vi "SPC_get_eeprom_data.vi"(8 "Error In":errorcluster, 10 "Module No":i16 min=0 max=31 step=1, 11 "DLL Path":path) -> (0 "Error Out":errorcluster, 2 "Module No":i16 min=0 max=7 step=1, 3 "DLL Path":path, 4 "Revision [U8]":u8[](array[numeric]), 5 "SPC EEPROM Data":T1={"module_type[16]"="                ", "serial_no[16]"="                ", "date[16]"="                ", "SPC adjust parameters"={"vrt1"=64, "vrt2"=128, "vrt3"=192, "dith_g"=128, "gain_1"=1.0, "gain_2"=1.0, "gain_4"=1.0, "gain_8"=1.0, "tac_r0"=1.0, "tac_r1"=1.0, "tac_r2"=1.0, "tac_r4"=1.0, "tac_r8"=1.0, "sync_div"=0}} {"SPC adjust parameters"."sync_div" min=0 max=2; "SPC adjust parameters"."tac_r8" format="%.2f"; "SPC adjust parameters"."tac_r4" format="%.2f"; "SPC adjust parameters"."tac_r2" format="%.2f"; "SPC adjust parameters"."tac_r1" format="%.2f"; "SPC adjust parameters"."tac_r0" format="%.2f"; "SPC adjust parameters"."gain_8" format="%.2f"; "SPC adjust parameters"."gain_4" format="%.2f"; "SPC adjust parameters"."gain_2" format="%.2f"; "SPC adjust parameters"."gain_1" format="%.2f"}, 6 "Revision":i16)   [LabVIEW 2023]
doc: "The structure \"eep_data\" is filled with the contents of EEPROM of SPC module ‘mod_no’. \nThe EEPROM contains production data and adjust parameters of the module. The structure \"SPC_EEP_Data\" is defined in the file spcm_def.h.\nNormally, the EEPROM data need not be read explicitly because the EEPROM is read during SPC_init and the module type information and the adjust values are taken into account when the SPC module registers are loaded.\n\ninfo@becker-hickl.com"
uses:
  SPC_Controls/SPC_eep_data.ctl
  SPC_Controls/SPC_adjust_para.ctl
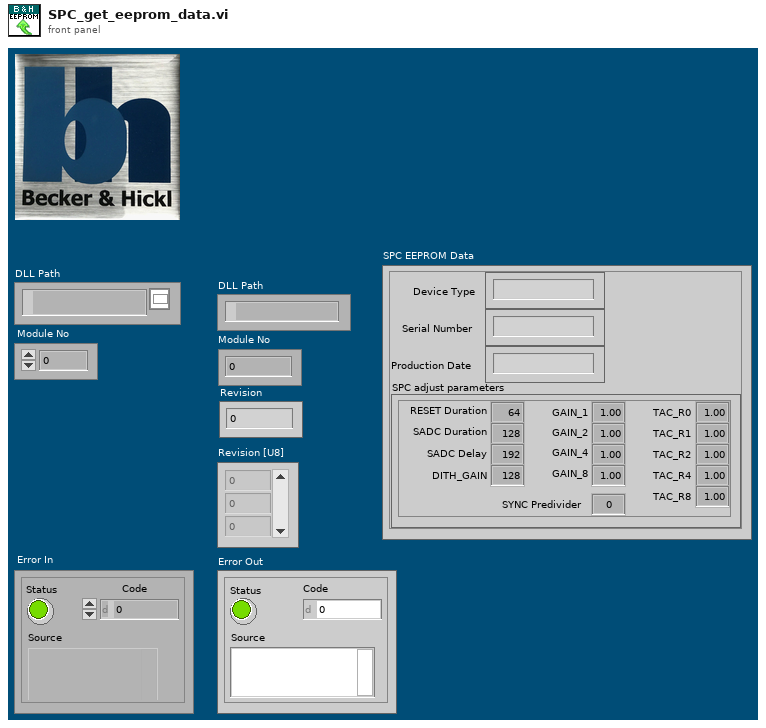
[diagram p1: front panel]
types:
  T1 = typedef "SPC_eep_data.ctl" = cluster{"module_type[16]":string, "serial_no[16]":string, "date[16]":string, "SPC adjust parameters":T2}
  T2 = typedef "SPC_adjust_para.ctl" = cluster{"vrt1":i16, "vrt2":i16, "vrt3":i16, "dith_g":i16, "gain_1":sgl, "gain_2":sgl, "gain_4":sgl, "gain_8":sgl, "tac_r0":sgl, "tac_r1":sgl, "tac_r2":sgl, "tac_r4":sgl, "tac_r8":sgl, "sync_div":i16}
  T3 = cluster{"[0]":u8, "[1]":u8, "[2]":u8, "[3]":u8, "[4]":u8, "[5]":u8, "[6]":u8, "[7]":u8, "[8]":u8, "[9]":u8, "[10]":u8, "[11]":u8, "[12]":u8, "[13]":u8, "[14]":u8, "[15]":u8}
  T4 = cluster{cluster{"[0]":u8, "[1]":u8, "[2]":u8, "[3]":u8, "[4]":u8, "[5]":u8, "[6]":u8, "[7]":u8, "[8]":u8, "[9]":u8, "[10]":u8, "[11]":u8, "[12]":u8, "[13]":u8, "[14]":u8, "[15]":u8}, cluster{"[0]":u8, "[1]":u8, "[2]":u8, "[3]":u8, "[4]":u8, "[5]":u8, "[6]":u8, "[7]":u8, "[8]":u8, "[9]":u8, "[10]":u8, "[11]":u8, "[12]":u8, "[13]":u8, "[14]":u8, "[15]":u8}, cluster{"[0]":u8, "[1]":u8, "[2]":u8, "[3]":u8, "[4]":u8, "[5]":u8, "[6]":u8, "[7]":u8, "[8]":u8, "[9]":u8, "[10]":u8, "[11]":u8, "[12]":u8, "[13]":u8, "[14]":u8, "[15]":u8}, "SPC adjust parameters":T2}
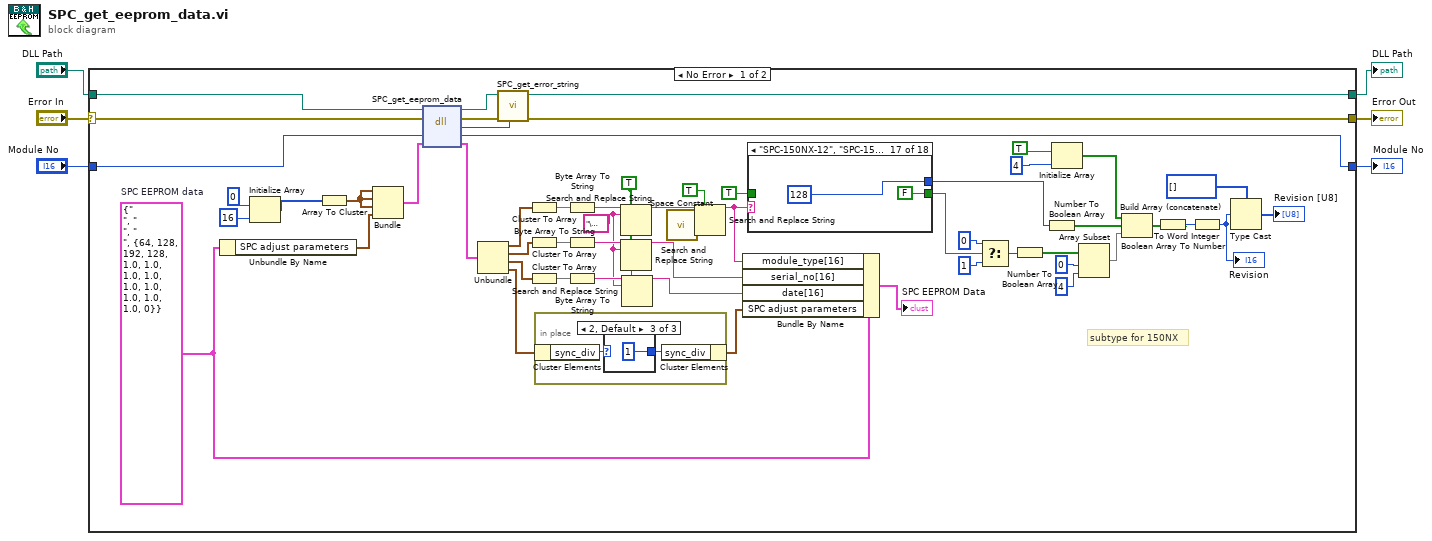
[diagram p0: block diagram]
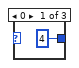
[diagram p2: hidden frame]
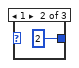
[diagram p3: hidden frame]
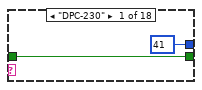
[diagram p4: hidden frame]
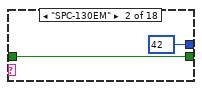
[diagram p5: hidden frame]
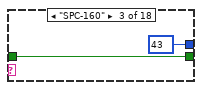
[diagram p6: hidden frame]
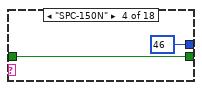
[diagram p7: hidden frame]
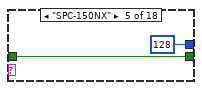
[diagram p8: hidden frame]
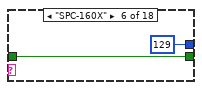
[diagram p9: hidden frame]
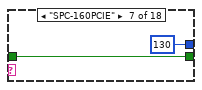
[diagram p10: hidden frame]
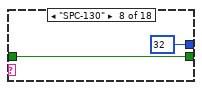
[diagram p11: hidden frame]
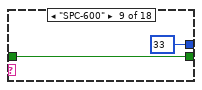
[diagram p12: hidden frame]
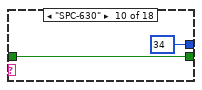
[diagram p13: hidden frame]
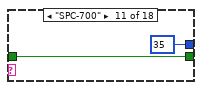
[diagram p14: hidden frame]
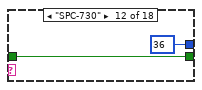
[diagram p15: hidden frame]
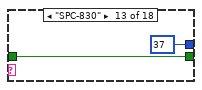
[diagram p16: hidden frame]
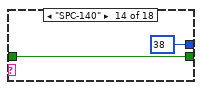
[diagram p17: hidden frame]
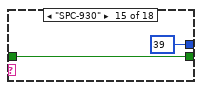
[diagram p18: hidden frame]
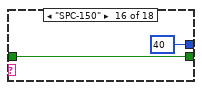
[diagram p19: hidden frame]
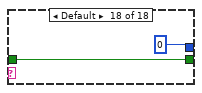
[diagram p20: hidden frame]
diagram:
  n1 = case shown="No Error" "Error In" {
    selector: "Error In" -> [w60 w106]
    tunnel: "DLL Path" -> [w59 w105]
    tunnel: [w53 w105] -> w4
    tunnel: [w55 w106] -> w3
    tunnel: "Module No" -> [w58 w104]
    tunnel: [w57 w104] -> w1
    frame No Error {
      w10 = TRUE ("replace all? (F)")
      w9 = "\u0000" ("search string")
      w62 = T1 {"module_type[16]"="                ", "serial_no[16]"="                ", "date[16]"="                ", "SPC adjust parameters"={"vrt1"=64, "vrt2"=128, "vrt3"=192, "dith_g"=128, "gain_1"=1.0, "gain_2"=1.0, "gain_4"=1.0, "gain_8"=1.0, "tac_r0"=1.0, "tac_r1"=1.0, "tac_r2"=1.0, "tac_r4"=1.0, "tac_r8"=1.0, "sync_div"=0}}  # SPC EEPROM data
      # "subtype for 150NX"
      n2 = Unbundle By Name(w62) -> ("SPC adjust parameters"=w30:T2)
      n3 = Initialize Array(u8 0, 16 ("RequiredStringLength")) -> (w26:u8[])
      n4 = Array To Cluster(array=w26) -> (cluster=w25:T3)
      n5 = Bundle(w25, w25, w25, "SPC adjust parameters"=w30) -> (w29:T4)  [unwired: 1 in]
      n6 = dll-call lib="C:/Program Files (x86)/BH/SPCM/DLL/spcm64.dll" fn="SPC_get_eeprom_data"(path in=w59, error in=w60, "mod_no"=w58, "EEPROM data"=w29) -> (path out=w54:path, error out=w56:errorcluster, "return type"=w52:i16, "mod_no"=w57:i16, "EEPROM data"=w51:T4)  [unwired: 1 in]
      n7 = Unbundle(w51) -> (w24:T3, w22:T3, w23:T3, "SPC adjust parameters"=w8:T2)
      n8 = call "SPC_get_error_string.vi"("ErrorID"=w52, "Error In"=w56, "DLL Path"=w54) -> ("Error Out"=w55:errorcluster, "DLL Path"=w53:path)  [unwired: 6 in, 1 out]
      n9 = Cluster To Array(cluster=w24) -> (array=w19:u8[])
      n10 = Cluster To Array(cluster=w22) -> (array=w21:u8[])
      n11 = Cluster To Array(cluster=w23) -> (array=w20:u8[])
      n12 = in-place {
        n13 = in-place-cluster #1(w8) -> ("sync_div"=w64:i16)
        n14 = case shown="2, Default" w64 {
          tunnel: [i16 4 ("sync_div") i16 2 ("sync_div") i16 1 ("sync_div")] -> w63
          frame 0 {
          }
          frame 1 {
          }
          frame 2, Default {
          }
        }
        n15 = in-place-cluster #1("sync_div"=w63) -> (w7:T2)
      }
      n16 = Byte Array To String(unsigned byte array=w19) -> (string=w16:string)
      n17 = Byte Array To String(unsigned byte array=w21) -> (string=w14:string)
      n18 = Byte Array To String(unsigned byte array=w20) -> (string=w12:string)
      n19 = Search and Replace String(replace all?=w10, input string=w16, search string=w9) -> (result string=w15:string)  [unwired: 5 in, 3 out]
      n20 = Search and Replace String(replace all?=w10, input string=w14, search string=w9) -> (result string=w13:string)  [unwired: 5 in, 3 out]
      n21 = Search and Replace String(replace all?=w10, input string=w12, search string=w9) -> (result string=w11:string)  [unwired: 5 in, 3 out]
      n22 = call <vilib>:"Space Constant.vi"() -> ("String"=w18:string)
      n23 = Search and Replace String(replace all?=TRUE ("replace all? (F)"), input string=w15, search string=w18) -> (result string=w37:string)  [unwired: 5 in, 3 out]
      n24 = Bundle By Name(cluster=w62, "module_type[16]"=w37, "serial_no[16]"=w13, "date[16]"=w11, "SPC adjust parameters"=w7) -> (→"SPC EEPROM Data":T1)
      n25 = case shown="\"SPC-150NX-12\", \"SPC-150NXX\"" w37 {
        tunnel: [u8 41 u8 42 u8 43 u8 46 u8 128 u8 129 u8 130 u8 32 u8 33 u8 34 u8 35 u8 36 u8 37 u8 38 u8 39 u8 40 u8 128 u8 0] -> w32
        tunnel: [w68 w70 w72 w74 w76 w78 w80 w82 w84 w86 w88 w90 w92 w94 w96 w98 FALSE w103] -> w49
        tunnel: TRUE -> [w68 w70 w72 w74 w76 w78 w80 w82 w84 w86 w88 w90 w92 w94 w96 w98 _ w103]
        frame "DPC-230" {
        }
        frame "SPC-130EM" {
        }
        frame "SPC-160" {
        }
        frame "SPC-150N" {
        }
        frame "SPC-150NX" {
        }
        frame "SPC-160X" {
        }
        frame "SPC-160PCIE" {
        }
        frame "SPC-130" {
        }
        frame "SPC-600" {
        }
        frame "SPC-630" {
        }
        frame "SPC-700" {
        }
        frame "SPC-730" {
        }
        frame "SPC-830" {
        }
        frame "SPC-140" {
        }
        frame "SPC-930" {
        }
        frame "SPC-150" {
        }
        frame "SPC-150NX-12", "SPC-150NXX" {
        }
        frame Default {
        }
      }
      n26 = Select(t=u8 0, s=w49, f=u8 1) -> (s? t:f=w31:u8)
      n27 = Number To Boolean Array(number=w31) -> (Boolean array=w42:bool[])
      n28 = Number To Boolean Array(number=w32) -> (Boolean array=w36:bool[])
      n29 = Initialize Array(TRUE, 4) -> (w33:bool[])
      n30 = Array Subset(array=w42, index=0, length=4) -> (w43:bool[])
      n31 = Build Array (concatenate)(w33, w36, w43) -> (w41:bool[])
      n32 = Boolean Array To Number(Boolean array=w41) -> (number=w46:u32)
      n33 = To Word Integer(number=w46) -> (16bit integer=w39:i16)
      "Revision" <- w39
      n34 = Type Cast(type=u8[] [], x=w39) -> (*(type *) &x=→"Revision [U8]":u8[])
    }
    frame Error {
    }
  }
  "DLL Path" <- w4
  "Error Out" <- w3
  "Module No" <- w1
